vi "append_numeric_value.vi"(1 "Numeric value":dbl=614.7, 2 "initial string":string) -> (0 "appended string":string)   [LabVIEW 2021]
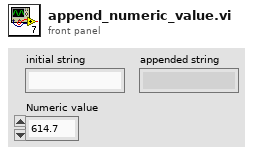
[diagram p1: front panel]
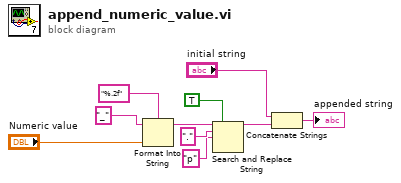
[diagram p0: block diagram]
diagram:
  n1 = Format Into String(format string="%.2f", initial string="_", "Numeric value") -> (resulting string=w7:string)  [unwired: 1 in, 1 out]
  n2 = Search and Replace String(replace all?=TRUE ("replace all? (F)"), input string=w7, search string=".", replace string="p" ("replace string (\"\")")) -> (result string=w2:string)  [unwired: 4 in, 3 out]
  n3 = Concatenate Strings("initial string", w2) -> (→"appended string":string)
